vi "User_Manage.vi"() -> ()   [LabVIEW 2020]
panel:
  in  "User List":i32(listbox)
  # "用户管理"
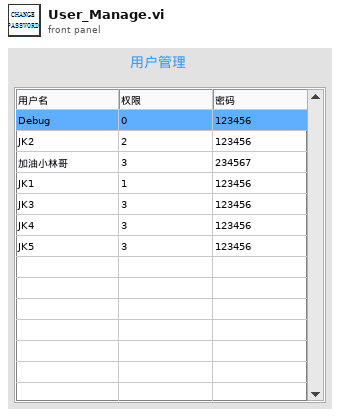
[diagram p1: front panel]
types:
  T1 = typedef "User_Info.ctl" = cluster{"Name":string, "Password":string, "User_Right":u16, "Debuger?":bool, "Manager?":bool, "User_Remember_Name":bool, "User_Remember_PW":bool, "User_Right_String":string, "Null?":bool, "Language":string}
  T2 = typedef "LVRowAndColumnTypeDef.ctl" = cluster{"Row":i32, "Column":i32}
  T3 = typedef "LVPoint32TypeDef.ctl" = cluster{"Horizontal":i32, "Vertical":i32}
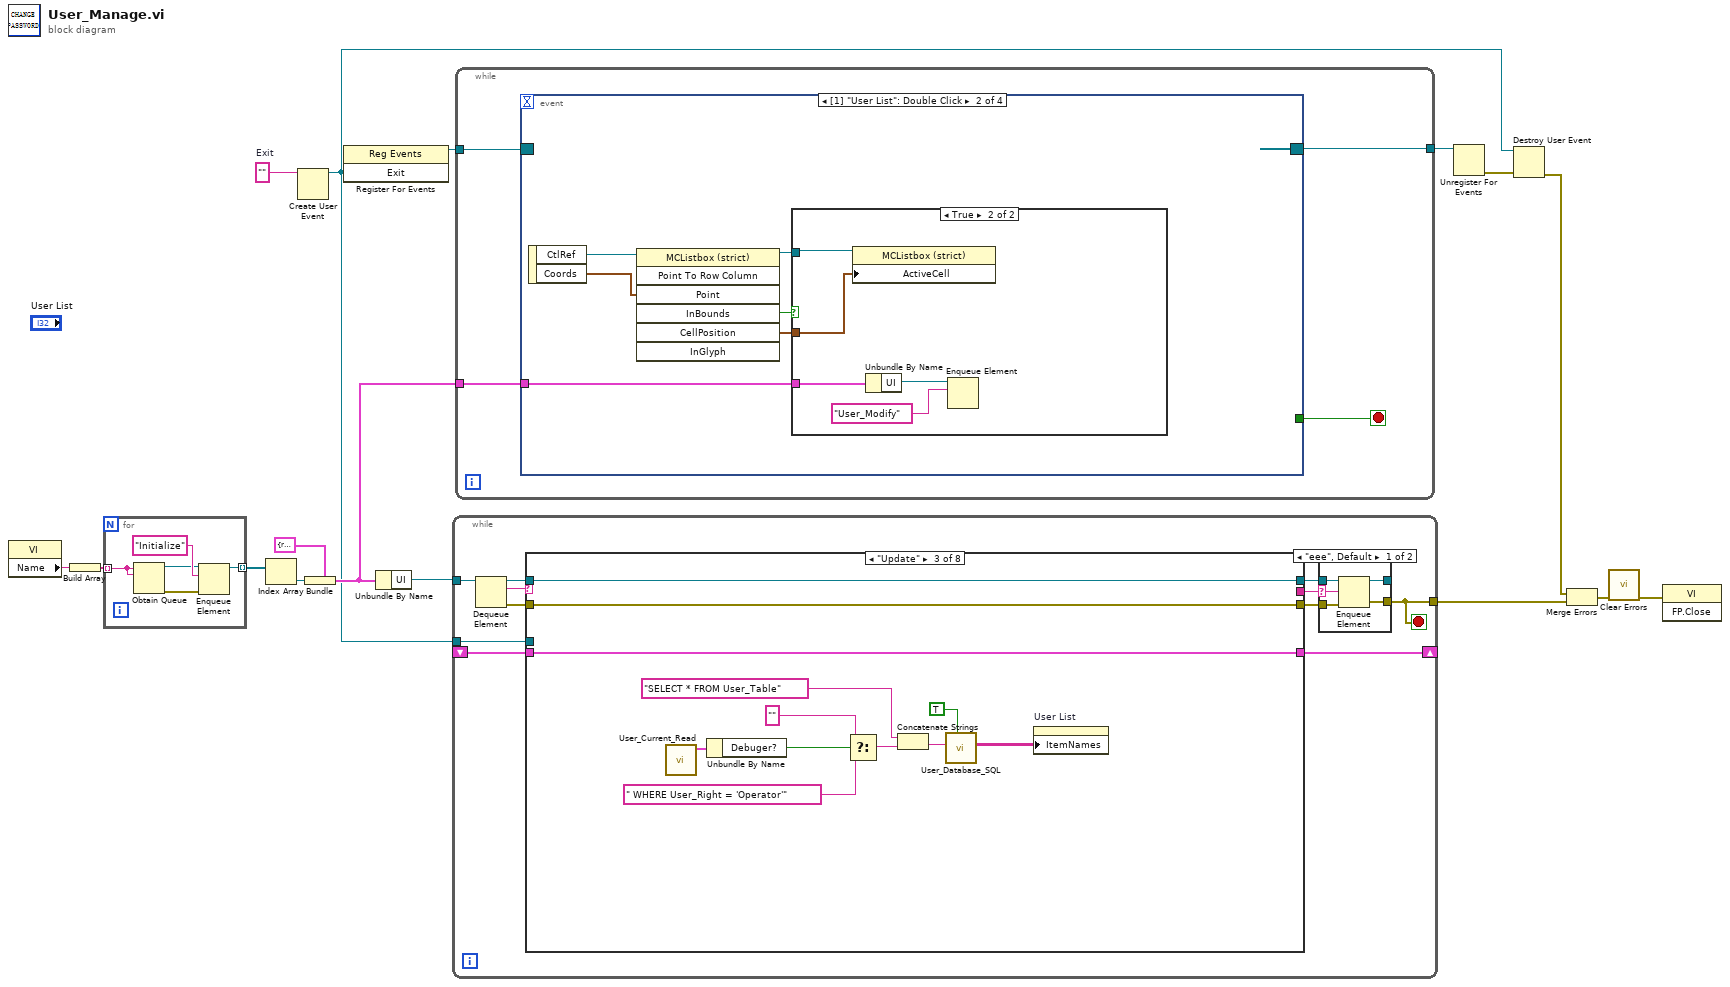
[diagram p0: block diagram]
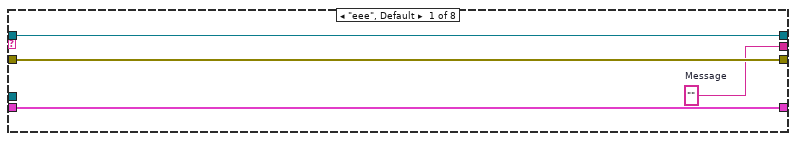
[diagram p3: hidden frame]
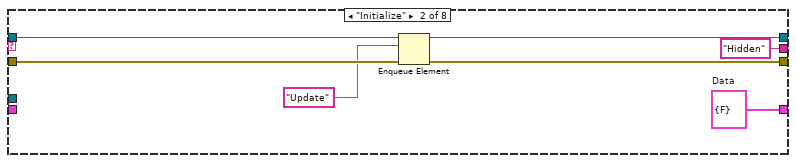
[diagram p4: hidden frame]
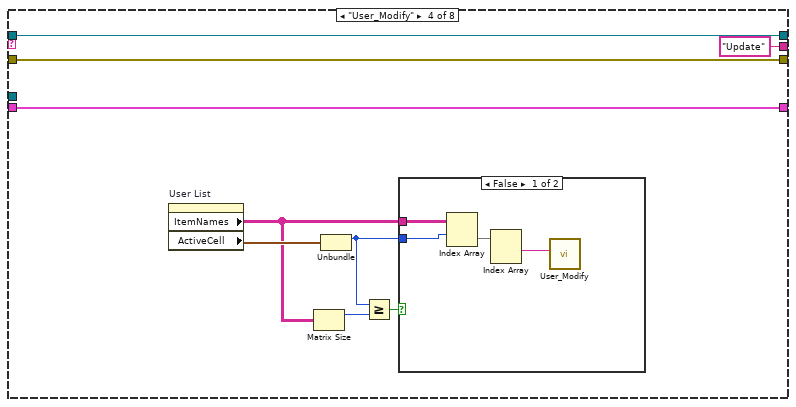
[diagram p5: hidden frame]
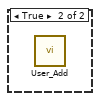
[diagram p6: hidden frame]
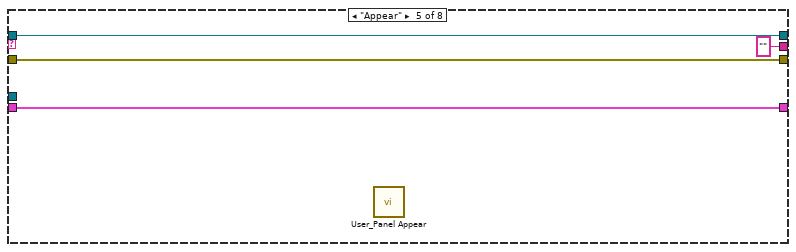
[diagram p7: hidden frame]
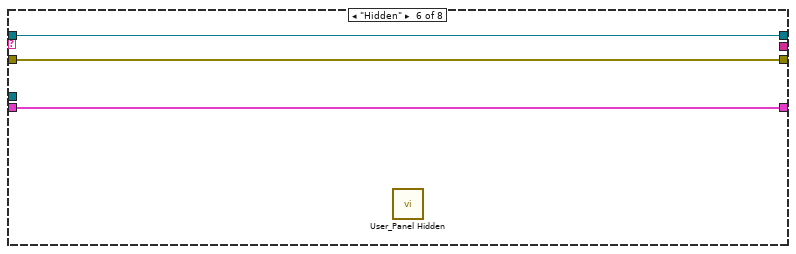
[diagram p8: hidden frame]
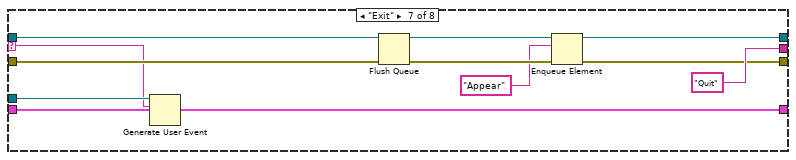
[diagram p9: hidden frame]
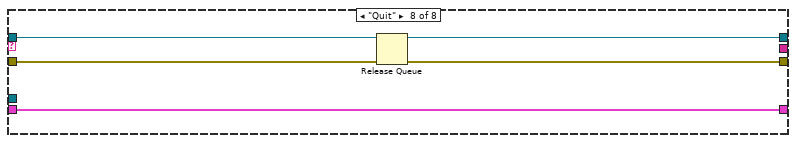
[diagram p10: hidden frame]
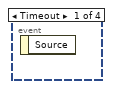
[diagram p11: hidden frame]
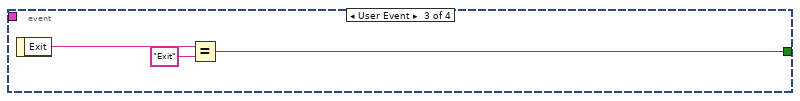
[diagram p13: hidden frame]
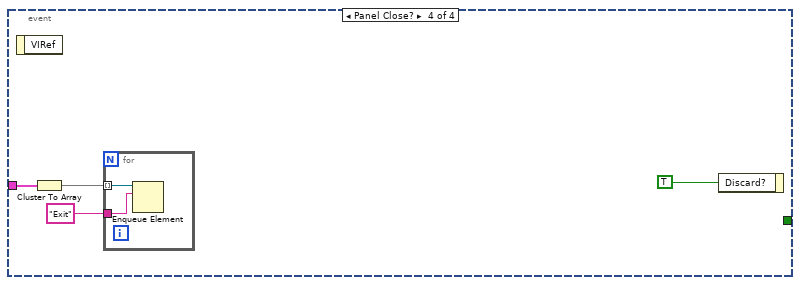
[diagram p14: hidden frame]
diagram:
  w2 = ""  # Exit
  n1 = property class="VI"() -> ("Name"=w12:string)  [unwired: 2 in, 2 out]
  n2 = Build Array(w12) -> (w13:string[])
  n3 = for {
    tunnel: w13 -> [w17] mode=indexing
    tunnel: [w18] -> w7 mode=indexing
    n4 = Obtain Queue(name (unnamed)=w17, element data type=w17) -> (queue out=w20:refnum<queue>, error out=w19:errorcluster)  [unwired: 3 in, 1 out]
    n5 = Enqueue Element(queue=w20, element="Initialize" ("元素"), error in (no error)=w19) -> (queue out=w18:refnum<queue>)  [unwired: 1 in, 2 out]
  }
  n6 = Index Array(array=w7) -> (element=w10:refnum<queue>)  [unwired: 1 in]
  n7 = Create User Event(user event datatype=w2) -> (user event=w6:refnum<user-event>)  [unwired: 1 in, 1 out]
  n8 = Bundle(cluster=cluster{"UI":refnum<queue>} {"UI"=refnum}, "UI"=w10) -> (w11:cluster{"UI":refnum<queue>})
  n9 = register-events(w6) -> (reference out=w3:refnum<event-registration>)  [unwired: 2 in, 1 out]
  n10 = Unbundle By Name(w11) -> ("UI"=w8:refnum<queue>)
  n11 = while {
    tunnel: w8 -> [w32]
    tunnel: [w22] -> w15
    shift-right: [w26] -> _
    shift-left: _ -> [w25]
    tunnel: w6 -> [w24]
    stop <- w22 stop-if-true
    n12 = Dequeue Element(queue=w32) -> (queue out=w31:refnum<queue>, element=w23:string, error out=w28:errorcluster)  [unwired: 2 in, 1 out]
    n13 = case shown="\"Update\"" w23 {
      selector: w23 -> [_ _ _ _ _ _ w88 _]
      tunnel: w31 -> [w43 w48 w62 w71 w79 w82 w91 w97]
      tunnel: [w43 w47 w62 w71 w79 w82 w84 w97] -> w30
      tunnel: [w42 w45 w61 w70 w78 w81 w85 w94] -> w29
      tunnel: w28 -> [w42 w46 w61 w70 w78 w81 w90 w96]
      tunnel: [w41 "Hidden" ("Message") _ "Update" ("Message") "" ("Message") _ "Quit" ("Message") _] -> w27
      tunnel: [w40 w50 w60 w69 w77 w80 w93 w95] -> w26
      tunnel: w25 -> [w40 _ w60 w69 w77 w80 w93 w95]
      tunnel: w24 -> [_ _ _ _ _ _ w89 _]
      frame "eee", Default {
        w41 = ""  # Message
      }
      frame "Initialize" {
        w50 = cluster{"Data":bool} {"Data"=FALSE}  # Data
        n14 = Enqueue Element(queue=w48, element="Update" ("Message"), error in (no error)=w46) -> (queue out=w47:refnum<queue>, error out=w45:errorcluster)  [unwired: 1 in, 1 out]
      }
      frame "Update" {
        n15 = call "User_Current_Read.vi"() -> ("User_Info"=w58:T1)  [unwired: 10 in, 1 out]
        n16 = Unbundle By Name(w58) -> ("Debuger?"=w54:bool)
        n17 = Select(t="" ("f"), s=w54, f=" WHERE User_Right = 'Operator'" ("SQL query")) -> (s? t:f=w52:string)
        n18 = Concatenate Strings("SELECT * FROM User_Table" ("SQL query"), w52) -> (w53:string)
        n19 = call "User_Database_SQL.vi"("Get Record"=TRUE, "SQL query"=w53) -> ("Record"=w51:string[][])  [unwired: 7 in, 2 out]
        n20 = property on="User List" class="MCListbox (strict)"("ItemNames"=w51) -> ()  [unwired: 2 in, 2 out]
      }
      frame "User_Modify" {
        n21 = property on="User List" class="MCListbox (strict)"() -> ("ItemNames"=w66:string[][], "ActiveCell"=w67:T2)  [unwired: 2 in, 2 out]
        n22 = Matrix Size(0:w66) -> (1:w64:i32)  [unwired: 1 out]
        n23 = Unbundle(w67) -> ("Row"=w65:i32)  [unwired: 1 out]
        n24 = Greater Or Equal?(x=w65, y=w64) -> (x >= y?=w63:bool)
        n25 = case shown="False" w63 {
          tunnel: w66 -> [w73 _]
          tunnel: w65 -> [w72 _]
          frame False {
            n26 = Index Array(array=w73, index (row)=w72) -> (element=w75:string[])  [unwired: 1 in]
            n27 = Index Array(array=w75) -> (element #1=w74:string)  [unwired: 2 in, 1 out]
            n28 = call "User_Modify.vi"("User_Name"=w74) -> ()  [unwired: 11 in]
          }
          frame True {
            n29 = call "User_Add.vi"() -> ()  [unwired: 11 in, 1 out]
          }
        }
      }
      frame "Appear" {
        n30 = call "User_Panel Appear.vi"() -> ()  [unwired: 11 in, 1 out]
      }
      frame "Hidden" {
        n31 = call "User_Panel Hidden.vi"() -> ()  [unwired: 11 in, 1 out]
      }
      frame "Exit" {
        n32 = Generate User Event(user event=w89, event data cluster=w88) -> ()  [unwired: 2 in, 2 out]
        n33 = Flush Queue(queue=w91, error in (no error)=w90) -> (queue out=w87:refnum<queue>, error out=w86:errorcluster)  [unwired: 1 out]
        n34 = Enqueue Element(queue=w87, element="Appear" ("元素"), error in (no error)=w86) -> (queue out=w84:refnum<queue>, error out=w85:errorcluster)  [unwired: 1 in, 1 out]
      }
      frame "Quit" {
        n35 = Release Queue(queue=w97, error in (no error)=w96) -> (error out=w94:errorcluster)  [unwired: 1 in, 2 out]
      }
    }
    n36 = case shown="\"eee\", Default" w27 {
      selector: w27 -> [w33 _]
      tunnel: w30 -> [w37 w39]
      tunnel: w29 -> [w36 w38]
      tunnel: [w35 w38] -> w22
      tunnel: [w34 w39] -> _
      frame "eee", Default {
        n37 = Enqueue Element(queue=w37, element=w33, error in (no error)=w36) -> (queue out=w34:refnum<queue>, error out=w35:errorcluster)  [unwired: 1 in, 1 out]
      }
      frame "" {
      }
    }
  }
  n38 = while {
    tunnel: w3 -> [w100]
    tunnel: [w99] -> w5
    tunnel: w11 -> [w98]
    stop <- w101 stop-if-true
    n39 = event shown="[1] \"User List\": Double Click" {
      selector: w100 -> [_ _ _ _]
      dyn-events: [_ _ _ _] -> w99
      timeout: _ -> [_ _ _ _]
      tunnel: [_ _ w114 _] -> w101
      tunnel: w98 -> [_ w102 _ w118]
      event Timeout {
        n40 = event-data() -> ()  [unwired: 1 in, 1 out]
      }
      event "User List": Double Click {
        n41 = event-data() -> ("CtlRef"=w107:refnum<vi>, "Coords"=w106:T3)  [unwired: 1 in]
        n42 = invoke class="MCListbox (strict)" method="Point To Row Column"(reference=w107, "Point"=w106) -> (reference out=w103:refnum<vi>, "InBounds"=w105:bool, "CellPosition"=w104:T2)  [unwired: 5 in, 4 out]
        n43 = case shown="True" w105 {
          tunnel: w104 -> [_ w111]
          tunnel: w103 -> [_ w112]
          tunnel: w102 -> [_ w110]
          frame False {
          }
          frame True {
            n44 = property class="MCListbox (strict)"(reference=w112, "ActiveCell"=w111) -> ()  [unwired: 1 in, 2 out]
            n45 = Unbundle By Name(w110) -> ("UI"=w109:refnum<queue>)
            n46 = Enqueue Element(queue=w109, element="User_Modify" ("元素")) -> ()  [unwired: 2 in, 3 out]
          }
        }
      }
      event User Event {
        n47 = event-data() -> ("Exit"=w115:string)  [unwired: 1 in]
        n48 = Equal?(x=w115, y="Exit") -> (x = y?=w114:bool)
      }
      event Panel Close? {
        n49 = event-data() -> ()  [unwired: 1 in, 1 out]
        n50 = Cluster To Array(cluster=w118) -> (array=w117:refnum<queue>[])
        n51 = for {
          tunnel: w117 -> [w121] mode=indexing
          tunnel: "Exit" ("元素") -> [w120]
          n52 = Enqueue Element(queue=w121, element=w120) -> ()  [unwired: 2 in, 3 out]
        }
        n53 = event-data("Discard?"=TRUE ("放弃？")) -> ()  [unwired: 1 in, 1 out]
      }
    }
  }
  n54 = Unregister For Events(event registration refnum=w5) -> (error out=w4:errorcluster)  [unwired: 1 in]
  n55 = Destroy User Event(user event=w6, error in=w4) -> (error out=w14:errorcluster)
  n56 = Merge Errors(w14, w15) -> (w16:errorcluster)
  n57 = call <vilib>:"Clear Errors.vi"("error in (no error)"=w16) -> ("error out"=w1:errorcluster)  [unwired: 5 in, 1 out]
  n58 = invoke class="VI" method="FP.Close"(error in=w1) -> ()  [unwired: 2 in, 3 out]
